vi "Low Pass Derivative.vi"(9 "Cutoff Freq":dbl, 10 "Sampling Freq":dbl, 11 "Input":dbl) -> (2 "Derivative Estimate":dbl)   [LabVIEW 2018]
uses:
  <vilib>/Analysis/3filter.llb/Filter Passband Type.ctl
  <vilib>/Analysis/NI_AALBase.lvlib
  <vilib>/ptbypt/NI_PtbyPt.lvlib
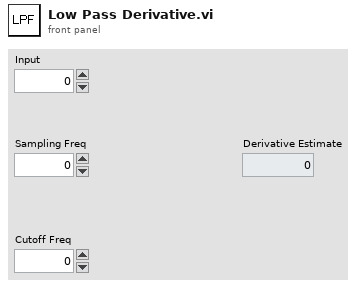
[diagram p1: front panel]
types:
  T1 = typedef "NI_AALBase.lvlib/Filter Passband Type.ctl" = enum32{"Lowpass", "Highpass", "Bandpass", "Bandstop"}
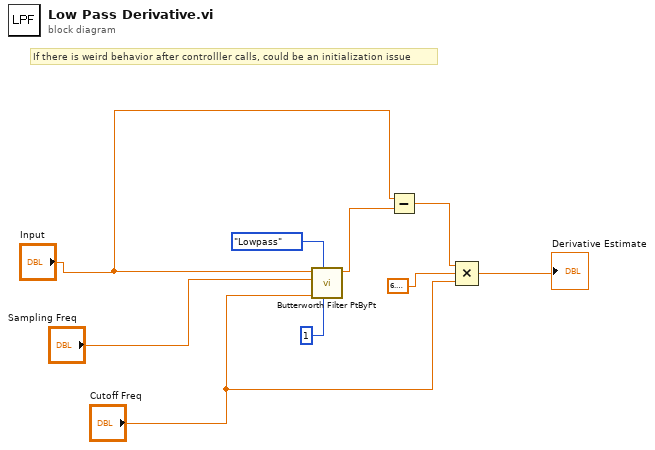
[diagram p0: block diagram]
diagram:
  # "If there is weird behavior after controlller calls, could be an initialization issue"
  n1 = call <vilib>:"Butterworth Filter PtByPt.vi"("order"=1, "filter type"=Filter_Passband_Type."Lowpass", "low cutoff freq: fl"="Cutoff Freq", "sampling freq: fs"="Sampling Freq", "x"="Input") -> ("Filtered x"=w5:dbl)  [unwired: 4 in, 1 out]
  n2 = Subtract(x="Input", y=w5) -> (x-y=w4:dbl)
  n3 = Compound Arithmetic op=MULTIPLY(w4, 6.283185307179586, "Cutoff Freq") -> (→"Derivative Estimate":dbl)
